vi "CRYProject Editor.vi"() -> ()   [LabVIEW 2013]
uses:
  <vilib>/Utility/miscctls.llb/LVBoundsTypeDef.ctl
  <vilib>/event_ctls.llb/eventvkey.ctl
  CRYProject Editor Global.vi
  CRYStepSetup/CRYStepSetup Global.vi
  CRYWindow/SubVI/CRYMain Sub Window Global.vi
  CRYCurveLibrary/Global/CRYCurve Library Global.vi
  CRYMainGlobal.vi
  CRYSystem/Task Sequence/CRYProject Run Control Global.vi
panel:
  out "OldPos":T1
  in  "StateOut":bool
  in  "Arg1":string
  out "RecentProjectLoad":i32
  out "EditFlag":bool
  in  "TS Name":u16(ring) items=["新建序列.cry"]
  in  "Add Step":bool
  in  "Expand/Collapse":bool caption="LegendShowOnOff"
  in  "ConfigureShowOnOff":bool caption="LegendShowOnOff"
  in  "Property seq":bool
  in  "Property step":bool
  in  "TitleShowOnOff":bool
  in  "Remove":bool
  in  "Move Down":bool
  in  "Move Up":bool
  in  "bWait":bool
  in  "TS Tree1":string(tree)
  in  "StepRemove":bool
  in  "StepLoad":bool
  in  "ProjectStateChange":bool
  in  "Load":bool
  in  "SequenceUpdate":bool
  in  "AllChange":bool
  in  "Insert":bool
  in  "Close All":bool
  in  "Close":bool
  in  "New":bool
  in  "Save":bool
  in  "Open":bool
  in  "Save As":bool
  in  "stop":bool
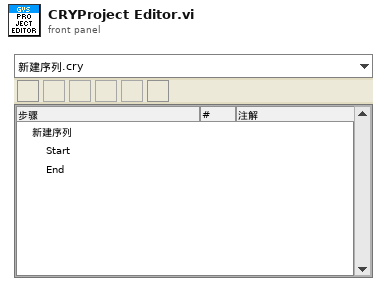
[diagram p1: front panel]
types:
  T1 = typedef "LVBoundsTypeDef.ctl" = cluster{"Width":u32, "Height":u32}
  T2 = cluster{"EventName":string, "Arg1":string, "Numeric":u16, "Numeric 2":u16, "AddSteps ":refnum<vi>, "Arg1 2":string, "Arg1 3":string, "Boolean":bool}
  T3 = typedef "eventvkey.ctl" = enum16{"ASCII", "Enter", "Return", "Shift", "Ctrl", "Alt", "Cmd", "Opt", "Caps", "NumLock", "Clear", "Break", "Up", "Down", "Left", "Right", "Insert", "Delete", "Home", "End", "PageUp", "PageDown", "Escape", "Help", "Pause", "ScrollLock", "F1", "F2", "F3", "F4", "F5", "F6", "F7", "F8", "F9", "F10", "F11", "F12", "F13", "F14", "F15", "F16", "F17", "F18", "F19", "F20", "F21", "F22", "F23", "F24", "Play", "VolumeUp", "VolumeDown", "Mute", "Two Byte Char"}
  T4 = enum16{"OK", "Yes", "YesNo", "YesNoCancel", "ReplaceAppend"}
  T5 = typedef "LVRectTypeDef.ctl" = cluster{"Left":i16, "Top":i16, "Right":i16, "Bottom":i16}
  T6 = typedef "LVPoint32TypeDef.ctl" = cluster{"Horizontal":i32, "Vertical":i32}
  T7 = typedef "CRYTS.ctl" = cluster{"No.TS":u16, "TS File Path":path, "TS Name":string, "EditStepName":string, "Steps":T8[], "New State":bool, "Change State":bool, "Flattened CurveLib Data":string, "Document Data":string, "EditStepNo":u16, "Operator Start File":string, "Sequence Type":string, "Sequence Language":string}
  T8 = typedef "CRYStep.ctl" = cluster{"No.VI":i32, "Category":string, "StepName":string, "Seq setup flattened":string, "Comment":string, "Steps config.":bool[], "Jump config":i32[], "Start":dbl, "Increment":dbl, "Name":string, "Unit":string, "Y data":u16, "Y prefix":string, "Y dB ref":dbl, "Y unit":string, "Repeat State Array":cluster{"Start":dbl, "Increment":dbl, "Count":i32, "Num":i32}[]}
  T9 = cluster{"Start":dbl, "Increment":dbl, "Count":i32, "Num":i32}[]
  T10 = cluster{"SourceRowNum":i32, "SourceCount":i32, "TargetRowNum":i32, "bResult":bool, "EditRowNum":i32}
  T11 = typedef "CRYProjectViewCluster.ctl" = cluster{"EventName":string, "Arg1":string, "Numeric":i32, "Proper VI No":i32, "AddSteps ":refnum<vi>, "Arg2":string, "Arg3":string, "Boolean":bool, "Mode":string, "Ref Variant":variant, "AllChangeFlg":bool}
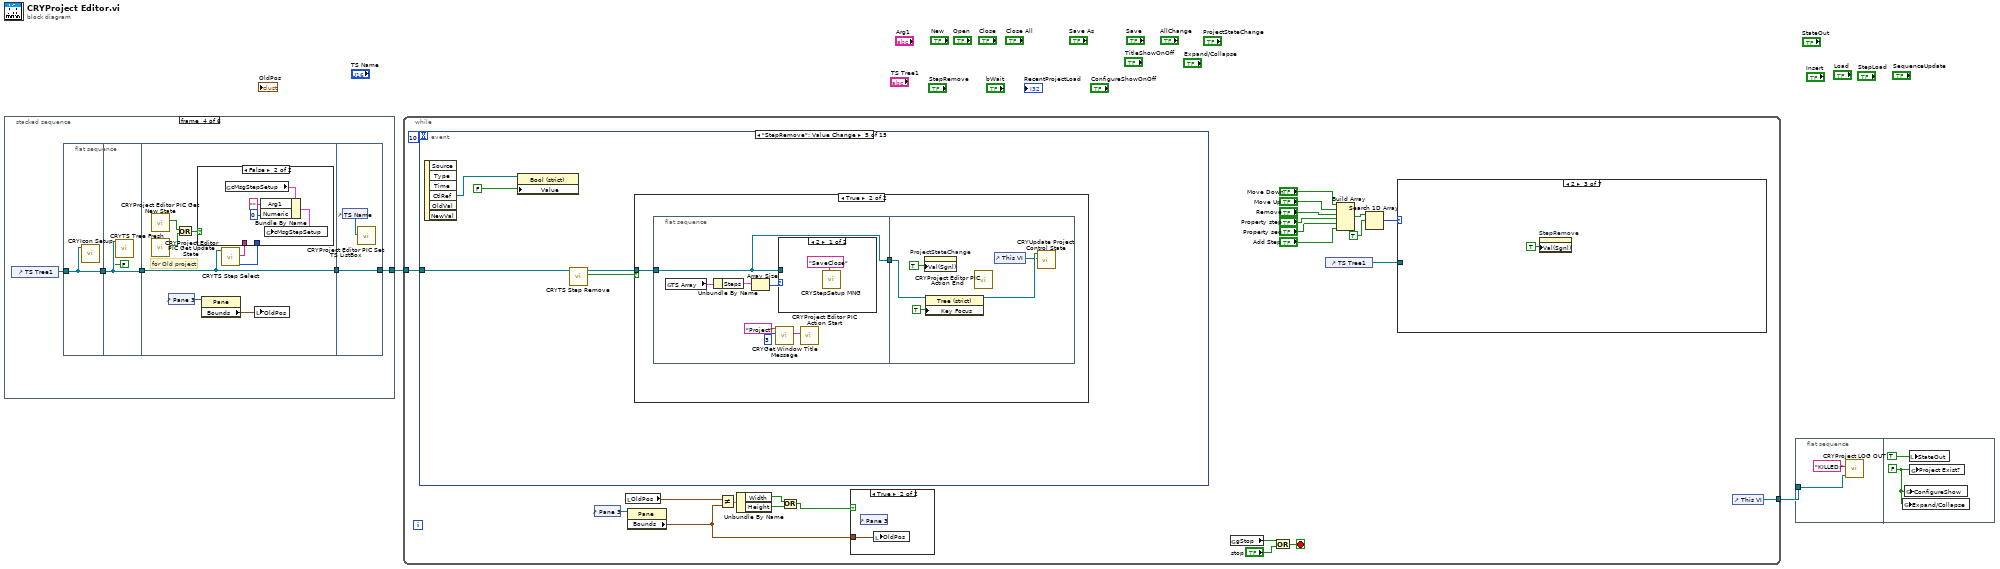
[diagram p0: block diagram]
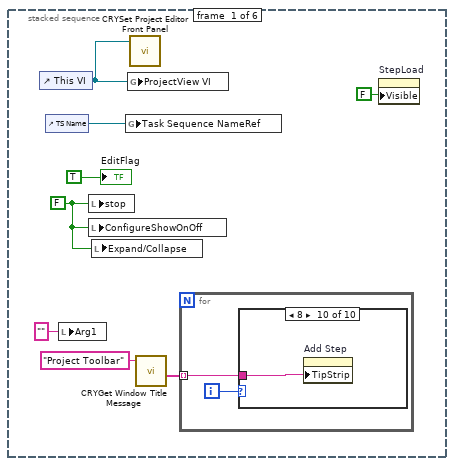
[diagram p2: hidden frame]
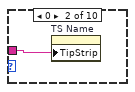
[diagram p4: hidden frame]
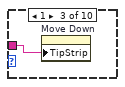
[diagram p5: hidden frame]
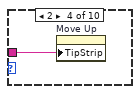
[diagram p6: hidden frame]
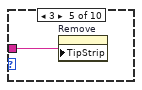
[diagram p7: hidden frame]
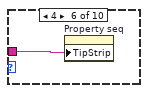
[diagram p8: hidden frame]
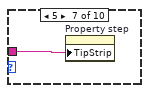
[diagram p9: hidden frame]
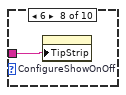
[diagram p10: hidden frame]
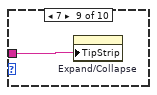
[diagram p11: hidden frame]
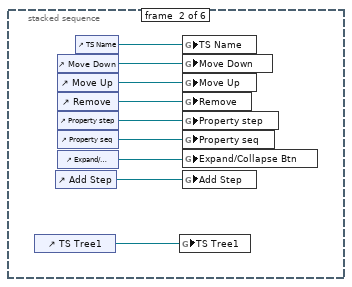
[diagram p12: hidden frame]
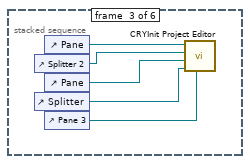
[diagram p13: hidden frame]
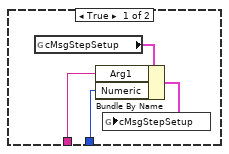
[diagram p14: hidden frame]
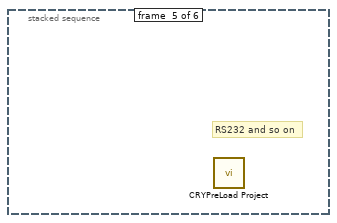
[diagram p15: hidden frame]
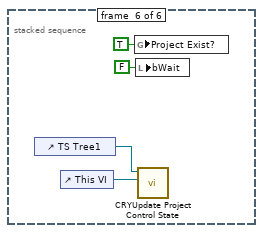
[diagram p16: hidden frame]
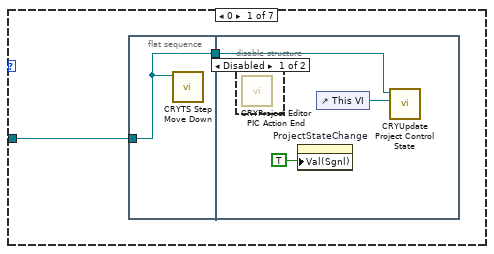
[diagram p17: hidden frame]
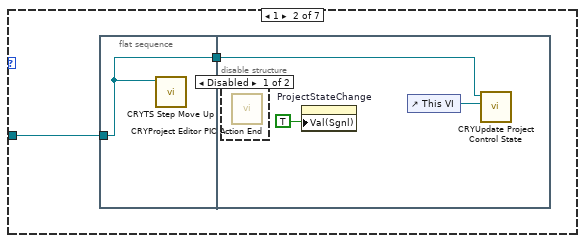
[diagram p19: hidden frame]
diagram:
  n1 = stacked-sequence {
    tunnel: [_ _ _ w36 _ _] -> w2
    frame #0 {
      w3 = FALSE ("stop")
      n2 = control-ref of="This VI"() -> (w4:refnum<vi>)
      n3 = control-ref of="TS Name"() -> (w10:refnum<vi>)
      n4 = local write "Arg1"("" ("Arg1")) -> ()
      n5 = local write "stop"(w3) -> ()
      n6 = local write "ConfigureShowOnOff"(w3) -> ()
      n7 = local write "Expand/Collapse"(w3) -> ()
      n8 = global write "CRYProject Editor Global.vi" "Task Sequence NameRef"(w10) -> ()
      n9 = global write "CRYProject Editor Global.vi" "ProjectView VI"(w4) -> ()
      n10 = call "CRYSet Project Editor Front Panel.vi"("Vi Ref"=w4) -> ()  [unwired: 11 in]
      n11 = call "CRYGet Window Title Message.vi"("Kind"="Project Toolbar") -> ("Tip Strip"=w5:string[])  [unwired: 5 in, 5 out]
      n12 = for {
        tunnel: w5 -> [w11] mode=indexing
        i -> [w12]
        n13 = case shown="8" w12 {
          tunnel: w11 -> [_ w13 w14 w15 w16 w17 w18 w19 w20 w21]
          frame Default {
          }
          frame 0 {
            n14 = property on="TS Name" class="Ring (strict)"("TipStrip"=w13) -> ()  [unwired: 2 in, 2 out]
          }
          frame 1 {
            n15 = property on="Move Down" class="Bool"("TipStrip"=w14) -> ()  [unwired: 2 in, 2 out]
          }
          frame 2 {
            n16 = property on="Move Up" class="Bool"("TipStrip"=w15) -> ()  [unwired: 2 in, 2 out]
          }
          frame 3 {
            n17 = property on="Remove" class="Bool"("TipStrip"=w16) -> ()  [unwired: 2 in, 2 out]
          }
          frame 4 {
            n18 = property on="Property seq" class="Bool"("TipStrip"=w17) -> ()  [unwired: 2 in, 2 out]
          }
          frame 5 {
            n19 = property on="Property step" class="Bool"("TipStrip"=w18) -> ()  [unwired: 2 in, 2 out]
          }
          frame 6 {
            n20 = property on="ConfigureShowOnOff" class="Bool (strict)"("TipStrip"=w19) -> ()  [unwired: 2 in, 2 out]
          }
          frame 7 {
            n21 = property on="Expand/Collapse" class="Bool (strict)"("TipStrip"=w20) -> ()  [unwired: 2 in, 2 out]
          }
          frame 8 {
            n22 = property on="Add Step" class="Bool"("TipStrip"=w21) -> ()  [unwired: 2 in, 2 out]
          }
        }
      }
      n23 = property on="StepLoad" class="Bool (strict)"("Visible"=FALSE) -> ()  [unwired: 2 in, 2 out]
      "EditFlag" <- TRUE ("EditFlag")
    }
    frame #1 {
      n24 = control-ref of="TS Tree1"() -> (w24:refnum<vi>)
      n25 = control-ref of="Add Step"() -> (w22:refnum<vi>)
      n26 = control-ref of="Move Down"() -> (w29:refnum<vi>)
      n27 = control-ref of="Move Up"() -> (w28:refnum<vi>)
      n28 = control-ref of="Remove"() -> (w27:refnum<vi>)
      n29 = control-ref of="Property step"() -> (w26:refnum<vi>)
      n30 = control-ref of="Property seq"() -> (w25:refnum<vi>)
      n31 = control-ref of="Expand/Collapse"() -> (w23:refnum<vi>)
      n32 = control-ref of="TS Name"() -> (w30:refnum<vi>)
      n33 = global write "CRYProject Editor Global.vi" "TS Tree1"(w24) -> ()
      n34 = global write "CRYProject Editor Global.vi" "TS Name"(w30) -> ()
      n35 = global write "CRYProject Editor Global.vi" "Move Down"(w29) -> ()
      n36 = global write "CRYProject Editor Global.vi" "Move Up"(w28) -> ()
      n37 = global write "CRYProject Editor Global.vi" "Remove"(w27) -> ()
      n38 = global write "CRYProject Editor Global.vi" "Property step"(w26) -> ()
      n39 = global write "CRYProject Editor Global.vi" "Property seq"(w25) -> ()
      n40 = global write "CRYProject Editor Global.vi" "Expand/Collapse Btn"(w23) -> ()
      n41 = global write "CRYProject Editor Global.vi" "Add Step"(w22) -> ()
    }
    frame #2 {
      n42 = control-ref of="Splitter 2"() -> (w34:refnum<vi>)
      n43 = control-ref of="Splitter"() -> (w32:refnum<vi>)
      n44 = control-ref of="Pane"() -> (w35:refnum<vi>)
      n45 = control-ref of="Pane"() -> (w33:refnum<vi>)
      n46 = control-ref of="Pane 3"() -> (w31:refnum<vi>)
      n47 = call "CRYInit Project Editor.vi"("Pane 3"=w31, "Splitter 2"=w32, "Pane 2"=w33, "Splitter 1"=w34, "Pane 1"=w35) -> ()  [unwired: 7 in]
    }
    frame #3 {
      n48 = control-ref of="TS Tree1"() -> (w38:refnum<vi>)
      n49 = flat-sequence {
        tunnel: w38 -> [w41]
        tunnel: [w41] -> w37
        tunnel: [w43] -> w39
        tunnel: w37 -> [w43]
        tunnel: w39 -> [w49]
        tunnel: [w49] -> w40
        tunnel: w40 -> [w61]
        tunnel: [w61] -> w36
        frame #0 {
          n50 = call "CRYIcon Setup.vi"("TS Tree In"=w41) -> ()  [unwired: 1 in, 8 out]
        }
        frame #1 {
          n51 = call "CRYTS Tree Fresh.vi"("SequenceTree"=w43, "Is Refresh?"=FALSE) -> ()  [unwired: 13 in, 1 out]
        }
        frame #2 {
          # "for Old project"
          n52 = call "CRYProject Editor PIC Get Update State.vi"() -> ("bChangeState"=w50:bool)  [unwired: 10 in, 1 out]
          n53 = call "CRYProject Editor PIC Get New State.vi"() -> ("bNewState"=w51:bool)  [unwired: 11 in]
          n54 = control-ref of="Pane 3"() -> (w45:refnum<vi>)
          n55 = Or(x=w51, y=w50) -> (x .or. y?=w48:bool)
          n56 = property class="Pane"(reference=w45) -> ("Bounds"=w44:T1)  [unwired: 1 in, 2 out]
          n57 = call "CRYTS Step Select.vi"("Tree reference In"=w49) -> ("nData_Out"=w46:i32, "sData_Out"=w47:string)  [unwired: 9 out]
          n58 = case shown="False" w48 {
            tunnel: w47 -> [w54 _]
            tunnel: w46 -> [w53 _]
            frame True {
              n59 = global read "CRYStepSetup Global.vi" "cMsgStepSetup"() -> (w55:T2)
              n60 = Bundle By Name(cluster=w55, "Arg1"=w54, "Numeric"=w53) -> (w52:T2)
              n61 = global write "CRYStepSetup Global.vi" "cMsgStepSetup"(w52) -> ()
            }
            frame False {
              n62 = global read "CRYStepSetup Global.vi" "cMsgStepSetup"() -> (w59:T2)
              n63 = Bundle By Name(cluster=w59, "Arg1"="", "Numeric"=u16 0) -> (w58:T2)
              n64 = global write "CRYStepSetup Global.vi" "cMsgStepSetup"(w58) -> ()
            }
          }
          n65 = local write "OldPos"(w44) -> ()
        }
        frame #3 {
          n66 = control-ref of="TS Name"() -> (w60:refnum<vi>)
          n67 = call "CRYProject Editor PIC Set TS ListBox.vi"("pRefTSListBox"=w60) -> ()  [unwired: 10 in, 1 out]
        }
      }
    }
    frame #4 {
      # "RS232 and so on"
      n68 = call "CRYPreLoad Project.vi"() -> ()  [unwired: 12 in]
    }
    frame #5 {
      n69 = control-ref of="TS Tree1"() -> (w62:refnum<vi>)
      n70 = control-ref of="This VI"() -> (w63:refnum<vi>)
      n71 = global write "CRYProject Editor Global.vi" "Project Exist?"(TRUE ("Project Exist?")) -> ()
      n72 = local write "bWait"(FALSE ("TreatingFlg")) -> ()
      n73 = call "CRYUpdate Project Control State.vi"("VI Ref"=w63, "RefTree In"=w62) -> ()  [unwired: 8 in, 2 out]
    }
  }
  n74 = while {
    tunnel: w2 -> [w88]
    tunnel: [w83] -> w1
    stop <- w84 stop-if-true
    n75 = event shown="[4] \"StepRemove\": Value Change" {
      selector: _ -> [_ _ _ _ _ _ _ _ _ _ _ _ _ _ _]
      dyn-events: _ -> [_ _ _ _ _ _ _ _ _ _ _ _ _ _ _]
      timeout: 10 -> [_ _ _ _ _ _ _ _ _ _ _ _ _ _ _]
      tunnel: w88 -> [_ w115 _ w133 w213 w240 w258 w264 w291 w296 w314 w316 w320 _ w356]
      event Timeout {
        n76 = event-data() -> ()  [unwired: 3 out]
      }
      event Pane Size {
        n77 = event-data() -> ("NewBnds"=w119:T5)  [unwired: 5 out]
        n78 = Unbundle By Name(w119) -> ("Right"=w118:i16, "Left"=w117:i16)  [unwired: 2 out]
        n79 = control-ref of="Splitter 2"() -> (w111:refnum<vi>)
        n80 = control-ref of="Splitter"() -> (w113:refnum<vi>)
        n81 = control-ref of="Pane"() -> (w110:refnum<vi>)
        n82 = control-ref of="Pane"() -> (w112:refnum<vi>)
        n83 = control-ref of="Pane 3"() -> (w114:refnum<vi>)
        n84 = Subtract(x=w118, y=w117) -> (x-y=w116:i16)
        n85 = call "CRYInit Project Editor.vi"("Pane 3"=w114, "Splitter 2"=w113, "Pane 2"=w112, "Splitter 1"=w111, "Pane 1"=w110) -> ()  [unwired: 7 in]
        n86 = disable-structure shown="Disabled" {
          disable-tunnel: w116 -> [w122 _]
          disable-tunnel: w115 -> [w120 _]
          frame Disabled {
            n87 = property on="Property Node" class="Tree (strict)"(reference=w120, "Width"=w122, "ActiveColNum"=0 ("Active Cell:Active Column Number")) -> ()  [unwired: 1 in, 2 out]
          }
          frame Enabled {
          }
        }
      }
      event "TS Tree1": Shortcut Menu Activation? {
        n88 = event-data() -> ("CtlRef"=w123:refnum<vi>, "MenuRef"=w128:refnum<k9>, "Coords"=w125:T6)  [unwired: 5 out]
        n89 = call "CRYGet Tree Click State.vi"("Coords"=w125, "Tree Ref In"=w123) -> ("Tag"=w124:string)  [unwired: 9 out]
        n90 = Not Equal?(x=w124, y="") -> (x != y?=w126:bool)
        n91 = case shown="True" w126 {
          tunnel: w128 -> [_ w132]
          tunnel: w123 -> [_ w130]
          tunnel: w125 -> [_ w131]
          frame False {
          }
          frame True {
            n92 = control-ref of="This VI"() -> (w129:refnum<vi>)
            n93 = call "CRYProject Popup Menu.vi"("Tree Reference In"=w130, "Coords In"=w131, "This VI"=w129, "Menu Ref In"=w132) -> ()  [unwired: 8 out]
          }
        }
        n94 = event-data() -> ()  [unwired: 1 in, 2 out]
      }
      event "TS Tree1": Shortcut Menu Selection (User) {
        n95 = event-data() -> ("CtlRef"=w134:refnum<vi>, "ItemTag"=w136:string, "Coords"=w135:T6)  [unwired: 6 out]
        n96 = case shown="\"STEP_RENAME\"" w136 {
          tunnel: w135 -> [_ _ w138 _ _ _ _]
          tunnel: w134 -> [_ w137 w139 _ _ _ w164]
          tunnel: w133 -> [_ _ _ w143 w146 _ _]
          frame "", Default {
          }
          frame "OPEN_SEQUENCE_CONFIGURE" {
            n97 = call "CRYStart Editor.vi"("Project Tree reference"=w137) -> ()  [unwired: 10 in, 1 out]
          }
          frame "OPEN_STEP_CONFIGURE" {
            n98 = call "CRYGet Tree Click State.vi"("Coords"=w138, "Tree Ref In"=w139) -> ()  [unwired: 10 out]
            n99 = call "CRYProject Tree Action Check.vi"("sOption"="Configure", "Project Tree reference"=w139) -> ("bResult"=w140:bool)  [unwired: 8 in, 1 out]
            n100 = case shown="True" w140 {
              tunnel: w139 -> [_ w142]
              frame False {
              }
              frame True {
                n101 = call "CRYConfigure Step.vi"("Project Tree reference"=w142) -> ()  [unwired: 10 in, 1 out]
              }
            }
          }
          frame "STEP_MOVE_DOWN" {
            n102 = flat-sequence {
              tunnel: w143 -> [w144]
              frame #0 {
                n103 = call "CRYTS Step Move Down.vi"("Sequence"=w144) -> ()  [unwired: 1 in, 10 out]
              }
              frame #1 {
                n104 = property on="ProjectStateChange" class="Bool (strict)"("Val(Sgnl)"=TRUE ("Value (Signaling)")) -> ()  [unwired: 2 in, 2 out]
              }
            }
          }
          frame "STEP_MOVE_UP" {
            n105 = flat-sequence {
              tunnel: w146 -> [w147]
              frame #0 {
                n106 = call "CRYTS Step Move Up.vi"("TreeRefereneIn"=w147) -> ()  [unwired: 1 in, 10 out]
              }
              frame #1 {
                n107 = property on="ProjectStateChange" class="Bool (strict)"("Val(Sgnl)"=TRUE ("Value (Signaling)")) -> ()  [unwired: 2 in, 2 out]
              }
            }
          }
          frame "STEP_DELETE" {
            n108 = property on="StepRemove" class="Bool (strict)"("Val(Sgnl)"=TRUE ("Value (Signaling)")) -> ()  [unwired: 2 in, 2 out]
          }
          frame "STEP_RENAME" {
            n109 = property on="Property Node" class="Tree (strict)"(reference=w164) -> (reference out=w168:refnum<vi>, "Value"=w163:string)  [unwired: 1 in, 1 out]
            n110 = global read "CRYProject Editor Global.vi" "TS Array"() -> (w157:T7)
            n111 = call "CRYGet Tree Step No.vi"("SequenceTree"=w164, "Active Item Tag"=w163) -> ("Active Cell String4"=w165:string)  [unwired: 12 in, 1 out]
            n112 = Decimal String To Number(string=w165) -> (number=w159:i32)  [unwired: 2 in, 1 out]
            n113 = Unbundle By Name(w157) -> ("Steps"=w156:T8[])
            n114 = property class="Tree (strict)"(reference=w168, "Active Item Tag"=w163, "ActiveColNum"=0 ("Active Cell:Active Column Number")) -> (reference out=w166:refnum<vi>, "Cell String"=w153:string)  [unwired: 1 in, 1 out]
            n115 = Index Array(array=w156, index=w159) -> (element=w158:T8)
            n116 = Unbundle By Name(w158) -> ("Repeat State Array"=w162:T9)
            n117 = Array Size(array=w162) -> (size(s)=w160:i32)
            n118 = for {
              N: w160 -> [_]
              shift-right: [w173] -> w151
              shift-left: "" ("decimal integer string") -> [w172]
              n119 = Concatenate Strings(w172, "     " ("decimal integer string")) -> (w173:string)
            }
            n120 = Match Pattern(string=w153, regular expression=w151) -> (before substring=w155:string, after substring=w154:string)  [unwired: 1 in, 2 out]
            n121 = Empty String/Path?(string/path=w155) -> (empty?=w150:bool)
            n122 = Select(t=w154, s=w150, f=w153) -> (s? t:f=w152:string)
            n123 = call "CRYGet Step Name Dialog.vi"("Step Name"=w152) -> ("Step Name Out"=w170:string, "Return Flag"=w169:bool)  [unwired: 9 in]
            n124 = case shown="True" w169 {
              tunnel: w166 -> [_ w187]
              tunnel: w170 -> [_ w176]
              tunnel: w163 -> [_ w186]
              tunnel: w159 -> [_ w185]
              tunnel: w158 -> [_ w184]
              tunnel: w157 -> [_ w182]
              tunnel: w156 -> [_ w183]
              tunnel: w150 -> [_ w181]
              tunnel: w151 -> [_ w180]
              frame False {
              }
              frame True {
                n125 = Select(t=w180, s=w181, f="") -> (s? t:f=w177:string)
                n126 = Concatenate Strings(w177, w176) -> (w178:string)
                n127 = flat-sequence {
                  tunnel: w187 -> [w201]
                  tunnel: w186 -> [w200]
                  tunnel: w185 -> [w191]
                  tunnel: w184 -> [w198]
                  tunnel: w183 -> [w197]
                  tunnel: w182 -> [w196]
                  tunnel: w178 -> [w195]
                  tunnel: w176 -> [w192]
                  tunnel: [w191] -> w175
                  tunnel: [w188] -> w174
                  tunnel: w175 -> [w209]
                  tunnel: w174 -> [w205]
                  frame #0 {
                    n128 = global read "CRYStepSetup Global.vi" "Step Setup Exist"() -> (w194:bool)
                    n129 = global read "CRYStepSetup Global.vi" "Step SubVI Ref"() -> (w193:refnum<vi>)
                    n130 = Bundle By Name(cluster=w198, "StepName"=w192) -> (w189:T8)
                    n131 = property class="Tree (strict)"(reference=w201, "Active Item Tag"=w200, "ActiveColNum"=0 ("Active Cell:Active Column Number"), "Cell String"=w195) -> ()  [unwired: 1 in, 2 out]
                    n132 = case shown="True" w194 {
                      tunnel: w193 -> [_ w204]
                      tunnel: w192 -> [_ w203]
                      frame False {
                      }
                      frame True {
                        n133 = property class="VI"(reference=w204, "Front Panel.Title"=w203) -> ()  [unwired: 1 in, 2 out]
                      }
                    }
                    n134 = Replace Array Subset(array=w197, new element=w189, index=w191) -> (w190:T8[])
                    n135 = Bundle By Name(cluster=w196, "Steps"=w190) -> (w199:T7)
                    n136 = global write "CRYProject Editor Global.vi" "TS Array"(w199) -> ()
                    n137 = Unbundle By Name(w189) -> ("No.VI"=w188:i32)
                  }
                  frame #1 {
                    n138 = global read "CRYCurve Library Global.vi" "Curve Library VI"() -> (w208:refnum<vi>)
                    n139 = call "CRYRename Data by Step Rename.vi"("Tree VI No."=w209) -> ()  [unwired: 11 in]
                    n140 = property on="ProjectStateChange" class="Bool (strict)"("Val(Sgnl)"=TRUE ("Value (Signaling)")) -> ()  [unwired: 2 in, 2 out]
                    n141 = call "CRYGet Numeric Reference.vi"("Label Name"="StepNameChange", "VI Refnum"=w208) -> ("Numeric Ref Out"=w206:refnum<vi>)  [unwired: 7 in, 2 out]
                    n142 = property class="DigNum"(reference=w206, "Val(Sgnl)"=w205) -> ()  [unwired: 1 in, 2 out]
                  }
                }
              }
            }
          }
        }
      }
      event "StepRemove": Value Change {
        n143 = event-data() -> ("CtlRef"=w214:refnum<vi>)  [unwired: 6 out]
        n144 = property on="Property Node" class="Bool (strict)"(reference=w214, "Value"=FALSE ("Remove")) -> ()  [unwired: 1 in, 2 out]
        n145 = call "CRYTS Step Remove.vi"("Tree Sequence"=w213) -> ("bResult"=w212:bool, "Tree Sequence Ref Out"=w211:refnum<vi>)  [unwired: 2 in, 7 out]
        n146 = case shown="True" w212 {
          tunnel: w211 -> [w218 w221]
          frame False {
            n147 = property class="Tree (strict)"(reference=w218, "Key Focus"=TRUE) -> (reference out=w216:refnum<vi>)  [unwired: 1 in, 1 out]
            n148 = control-ref of="This VI"() -> (w217:refnum<vi>)
            n149 = call "CRYUpdate Project Control State.vi"("VI Ref"=w217, "RefTree In"=w216) -> ()  [unwired: 8 in, 2 out]
          }
          frame True {
            n150 = flat-sequence {
              tunnel: w221 -> [w225]
              tunnel: [w225] -> w220
              tunnel: w220 -> [w234]
              frame #0 {
                n151 = global read "CRYProject Editor Global.vi" "TS Array"() -> (w223:T7)
                n152 = Unbundle By Name(w223) -> ("Steps"=w224:T8[])
                n153 = Array Size(array=w224) -> (size(s)=w222:i32)
                n154 = call "CRYGet Window Title Message.vi"("No"=3 ("Error No"), "Kind"="Project") -> ("Unicode String"=w227:string)  [unwired: 4 in, 5 out]
                n155 = case shown="2" w222 {
                  tunnel: w225 -> [_ w231]
                  frame 2 {
                    n156 = call "CRYStepSetup MNG.vi"("sAction"="SaveClose") -> ()  [unwired: 9 in, 2 out]
                  }
                  frame Default {
                    n157 = call "CRYTS Step Select.vi"("Tree reference In"=w231) -> ("nData_Out"=w232:i32, "sData_Out"=w233:string)  [unwired: 9 out]
                    n158 = call "CRYStep Setup Replace.vi"("sOption Etc"="StepRemove" ("sOption"), "Current Step Setup VI No"=w232, "Category"=w233) -> ()  [unwired: 1 in, 8 out]
                  }
                }
                n159 = call "CRYProject Editor PIC Action Start.vi"("sData"=w227) -> ()  [unwired: 11 in]
              }
              frame #1 {
                n160 = property on="ProjectStateChange" class="Bool (strict)"("Val(Sgnl)"=TRUE ("Value (Signaling)")) -> ()  [unwired: 2 in, 2 out]
                n161 = property class="Tree (strict)"(reference=w234, "Key Focus"=TRUE) -> (reference out=w238:refnum<vi>)  [unwired: 1 in, 1 out]
                n162 = call "CRYProject Editor PIC Action End.vi"() -> ()  [unwired: 12 in]
                n163 = control-ref of="This VI"() -> (w237:refnum<vi>)
                n164 = call "CRYUpdate Project Control State.vi"("VI Ref"=w237, "RefTree In"=w238) -> ()  [unwired: 8 in, 2 out]
              }
            }
          }
        }
      }
      event "Expand/Collapse": Value Change {
        n165 = event-data() -> ("NewVal"=w239:bool)  [unwired: 6 out]
        n166 = flat-sequence {
          tunnel: [w245] -> w243
          tunnel: w240 -> [w245]
          tunnel: w239 -> [w244]
          tunnel: [w250] -> w242
          tunnel: [w248] -> w241
          tunnel: w243 -> [w246]
          tunnel: w242 -> [w252]
          tunnel: w241 -> [w251]
          frame #0 {
            n167 = global write "CRYProject Editor Global.vi" "Expand/Collapse"(w244) -> ()
          }
          frame #1 {
            n168 = call "CRYCalculation TS Tree RowNum.vi"("Tree Task SequenceIn"=w246, "sOption"="Step Configure") -> ("DispInfo Cluster Out"=w249:T10, "Tree Task Sequence Out"=w250:refnum<vi>)  [unwired: 7 in, 5 out]
            n169 = Unbundle By Name(w249) -> ("EditRowNum"=w248:i32)
          }
          frame #2 {
            n170 = call "CRYTS Tree Fresh.vi"("SequenceTree"=w252, "Edit Index"=w251, "Is Refresh?"=FALSE) -> ()  [unwired: 12 in, 1 out]
          }
        }
      }
      event "Save As": Value Change {
        w259 = 0 ("Active Cell:Active Column Number")
        n171 = event-data() -> ()  [unwired: 7 out]
        n172 = control-ref of="TS Name"() -> (w261:refnum<vi>)
        n173 = property on="Property Node" class="Tree (strict)"(reference=w258, "Active Item Row Number"=w259, "ActiveColNum"=w259) -> (reference out=w260:refnum<vi>, "Active Item Tag"=w254:string)  [unwired: 1 in, 1 out]
        n174 = call "CRYProject Editor PIC Set TS ListBox.vi"("pRefTSListBox"=w261) -> ("TS Name Out"=w256:string)  [unwired: 10 in]
        n175 = Match Pattern(string=w256, regular expression=".cry") -> (before substring=w255:string)  [unwired: 1 in, 3 out]
        n176 = property on="Property Node" class="Tree (strict)"(reference=w260, "Active Item Tag"=w254, "Cell String"=w255) -> ()  [unwired: 1 in, 2 out]
      }
      event "TS Tree1": Double Click {
        n177 = event-data() -> ("Coords"=w263:T6, "Tag"=w265:string)  [unwired: 8 out]
        n178 = call "CRYGet Tree Click State.vi"("Coords"=w263, "Tree Ref In"=w264) -> ("In Bounds?"=w262:bool)  [unwired: 4 in, 5 out]
        n179 = case shown="True" w262 {
          tunnel: w265 -> [_ w268]
          tunnel: w264 -> [_ w267]
          tunnel: w263 -> [_ w266]
          frame False {
          }
          frame True {
            n180 = flat-sequence {
              tunnel: w267 -> [w273]
              tunnel: [w273] -> w271
              tunnel: [w275] -> w270
              tunnel: w266 -> [w275]
              tunnel: w268 -> [w274]
              tunnel: [w274] -> w269
              tunnel: w271 -> [w279]
              tunnel: w270 -> [w281]
              tunnel: w269 -> [w278]
              frame #0 {
                n181 = global read "CRYMainGlobal.vi" "Access Level"() -> (w272:enum16{"Engineer", "Technician", "Operator"})
                n182 = case shown="\"Engineer\"" w272 {
                  tunnel: w273 -> [w276 _]
                  frame "Engineer" {
                    n183 = control-ref of="This VI"() -> (w277:refnum<vi>)
                    n184 = call "CRYUpdate Project Control State.vi"("VI Ref"=w277, "RefTree In"=w276) -> ()  [unwired: 8 in, 2 out]
                  }
                  frame "Operator", Default {
                  }
                }
              }
              frame #1 {
                n185 = call "CRYProject Tree Action Check.vi"("tag"=w278, "Coords In"=w281, "sOption"="Tree DblClick", "Project Tree reference"=w279) -> ("Type Out"=w280:string, "bResult"=w282:bool)  [unwired: 6 in]
                n186 = case shown="True" w282 {
                  tunnel: w280 -> [_ w285]
                  tunnel: w279 -> [_ w284]
                  frame False {
                  }
                  frame True {
                    n187 = case shown="\"main\"" w285 {
                      tunnel: w284 -> [_ w286 w287 _]
                      frame Default {
                      }
                      frame "Seq Config" {
                        n188 = call "CRYStart Editor.vi"("Project Tree reference"=w286) -> ()  [unwired: 10 in, 1 out]
                      }
                      frame "Step Config" {
                        n189 = call "CRYConfigure Step.vi"("Project Tree reference"=w287) -> ()  [unwired: 10 in, 1 out]
                      }
                      frame "main" {
                        n190 = call "CRYPreUpdate Sequence.vi"("EventName"="StepLoadFromProject", "AllChangeFlg"=TRUE) -> ()  [unwired: 14 in]
                      }
                    }
                  }
                }
              }
            }
          }
        }
      }
      event "TS Tree1": Mouse Down {
        n191 = event-data() -> ()  [unwired: 9 out]
        n192 = global read "CRYMainGlobal.vi" "Access Level"() -> (w290:enum16{"Engineer", "Technician", "Operator"})
        n193 = case shown="\"Technician\", Default" w290 {
          tunnel: w291 -> [w292 _]
          frame "Engineer" {
            n194 = control-ref of="This VI"() -> (w293:refnum<vi>)
            n195 = call "CRYUpdate Project Control State.vi"("VI Ref"=w293, "RefTree In"=w292) -> ()  [unwired: 8 in, 2 out]
            n196 = local write "EditFlag"(TRUE ("EditFlag")) -> ()
          }
          frame "Technician", Default {
          }
        }
      }
      event "TS Tree1": Key Down {
        n197 = event-data() -> ("VKey"=w297:T3)  [unwired: 10 out]
        n198 = global read "CRYMainGlobal.vi" "Access Level"() -> (w295:enum16{"Engineer", "Technician", "Operator"})
        n199 = case shown="\"Technician\", Default" w295 {
          tunnel: w297 -> [w299 _]
          tunnel: w296 -> [w298 _]
          frame "Engineer" {
            n200 = flat-sequence {
              tunnel: w299 -> [w303]
              tunnel: [w303] -> w300
              tunnel: w298 -> [w302]
              tunnel: w300 -> [w306]
              frame #0 {
                n201 = control-ref of="This VI"() -> (w301:refnum<vi>)
                n202 = call "CRYUpdate Project Control State.vi"("VI Ref"=w301, "RefTree In"=w302) -> ()  [unwired: 8 in, 2 out]
              }
              frame #1 {
                n203 = Equal?(x=w306, y=eventvkey."Delete" ("VKey")) -> (x = y?=w304:bool)
                n204 = case shown="True" w304 {
                  frame False {
                  }
                  frame True {
                    n205 = property on="StepRemove" class="Bool (strict)"("Val(Sgnl)"=TRUE ("Value (Signaling)")) -> ()  [unwired: 2 in, 2 out]
                  }
                }
              }
            }
          }
          frame "Technician", Default {
            n206 = call "CRYGet Error Message.vi"("Kind"="Step Setup") -> ("Window Title"=w310:string)  [unwired: 5 in, 5 out]
            n207 = call "CRYGet Access Level Message.vi"() -> ("Multibyte string"=w308:string)  [unwired: 11 in]
            n208 = call "CRYMessage Dialog.vi"("Window Title"=w310, "YesNoCancel"=T4."OK", "Message Content"=w308) -> ()  [unwired: 7 in, 2 out]
          }
        }
      }
      event "TS Tree1": event type 3.0.x80000011; "TS Tree1": Item Open? {
        n209 = event-data() -> ("Tag"=w315:string)  [unwired: 5 out]
        n210 = invoke class="Tree (strict)" method="Double Click"(reference=w314) -> ("Double Click"=w313:string)  [unwired: 2 in, 2 out]
        n211 = Equal?(x=w315, y=w313) -> (x = y?=w312:bool)
        n212 = event-data("Discard?"=w312) -> ()  [unwired: 1 in, 1 out]
      }
      event "TS Tree1": event #0x1e; "TS Tree1": Item Close {
        n213 = event-data() -> ()  [unwired: 6 out]
        n214 = control-ref of="This VI"() -> (w317:refnum<vi>)
        n215 = local write "EditFlag"(FALSE ("EditFlag")) -> ()
        n216 = call "CRYUpdate Project Control State.vi"("VI Ref"=w317, "RefTree In"=w316) -> ()  [unwired: 8 in, 2 out]
      }
      event "TS Name": Value Change {
        n217 = event-data() -> ("CtlRef"=w322:refnum<vi>, "OldVal"=w319:u16)  [unwired: 5 out]
        n218 = property on="TS Name" class="Ring (strict)"() -> ("RingText.Text"=w323:string)  [unwired: 2 in, 2 out]
        n219 = flat-sequence {
          tunnel: w319 -> [w326]
          tunnel: w323 -> [w328]
          tunnel: [w328] -> w321
          tunnel: w322 -> [w327]
          tunnel: w320 -> [w324]
          tunnel: w321 -> [w329]
          frame #0 {
            n220 = property class="Ring (strict)"(reference=w327, "Value"=w326) -> ()  [unwired: 1 in, 2 out]
            n221 = control-ref of="This VI"() -> (w325:refnum<vi>)
            n222 = call "CRYUpdate Project Control State.vi"("VI Ref"=w325, "RefTree In"=w324) -> ()  [unwired: 8 in, 2 out]
          }
          frame #1 {
            n223 = global read "CRYProject Editor Global.vi" "TS Array"() -> (w331:T7)
            n224 = Unbundle By Name(w331) -> ("TS File Path"=w333:path)
            n225 = Path To String(path=w333) -> (string=w334:string)
            n226 = Concatenate Strings(w334, "\\" ("string"), w329) -> (w332:string)
            n227 = call "CRYProject Editor PIC Send Event to Main.vi"("nData"=0, "sData"=w332, "sEventName"="OpenProjectFullPath") -> ()  [unwired: 9 in]
          }
          frame #2 {
            n228 = call "CRYProject Editor PIC Action End.vi"() -> ()  [unwired: 12 in]
          }
        }
      }
      event "ProjectStateChange": Value Change {
        n229 = event-data() -> ()  [unwired: 7 out]
        n230 = global read "CRYProject Editor Global.vi" "bProjectLoaded"() -> (w342:bool)
        n231 = global read "CRYMainGlobal.vi" "Sequence Generator"() -> (w338:bool)
        n232 = global read "CRYProject Run Control Global.vi" "RunState"() -> (w341:bool)
        n233 = global read "CRYMainGlobal.vi" "Quick Lunch"() -> (w339:bool)
        n234 = Or(x=w339, y=w338) -> (x .or. y?=w337:bool)
        n235 = Compound Arithmetic op=AND(w342, invert w341, invert w337) -> (w340:bool)
        n236 = case shown="True" w340 {
          frame False {
          }
          frame True {
            n237 = global read "CRYProject Editor Global.vi" "TS Array"() -> (w345:T7)
            n238 = Unbundle By Name(w345) -> ("Change State"=w344:bool)
            n239 = case shown="False" w344 {
              selector: w344 -> [w352 w353]
              tunnel: [w352 w353] -> w343
              frame True {
              }
              frame False {
                n240 = call "CRYProject Editor PIC Change State.vi"("bChangeState"=TRUE ("Change State")) -> ()  [unwired: 11 in]
              }
            }
            n241 = flat-sequence {
              tunnel: w343 -> [_]
              frame #0 {
                n242 = global read "CRYMain Sub Window Global.vi" "Main Menu Refnum"() -> (w349:refnum<k9>)
                n243 = call "CRYMenu Language Set.vi"("sID"="FILE_SAVE") -> ("sMultibyte_Out"=w350:string, "sID_Out"=w351:string)  [unwired: 7 in, 2 out]
                n244 = Set Menu Item Info(6:FALSE ("checked"), 7:w351, 9:TRUE ("enabled"), 10:w350, 11:w349) -> ()  [unwired: 1 in, 3 out]
              }
            }
          }
        }
      }
      event "AllChange": Value Change {
        n245 = event-data() -> ()  [unwired: 7 out]
        n246 = local read "bWait"() -> (w355:bool)
        n247 = case shown="False" w355 {
          tunnel: w356 -> [w362 _]
          frame False {
            n248 = flat-sequence {
              tunnel: w362 -> [w366]
              tunnel: [w366] -> w361
              tunnel: [w372] -> w364
              tunnel: [w371] -> w363
              tunnel: w361 -> [w370]
              tunnel: [w369] -> w358
              tunnel: [w368] -> w357
              tunnel: w364 -> [w517]
              tunnel: w363 -> [w520]
              tunnel: [w517] -> w360
              tunnel: [w516] -> w359
              tunnel: w358 -> [_]
              tunnel: w357 -> [_]
              tunnel: w360 -> [w530]
              tunnel: w359 -> [w529]
              frame #0 {
                n249 = local write "bWait"(TRUE ("Project Exist?")) -> ()
              }
              frame #1 {
                n250 = call "CRYPull Data From ProjectViewCluster Array.vi"() -> ("Is Remain ?"=w372:bool, "ProjectViewCluster Out"=w371:T11)  [unwired: 10 in]
                n251 = global read "CRYMainGlobal.vi" "Access Level"() -> (w367:enum16{"Engineer", "Technician", "Operator"})
                n252 = Unbundle By Name(w371) -> ("EventName"=w368:string, "Arg1"=w374:string, "Proper VI No"=w373:i32)
                n253 = case shown="\"StepLoadFromProject\"" w368 {
                  tunnel: w370 -> [w375 w379 w388 w394 w406 w424 w441 w479 w480 w481 w482 w483 w490 w504]
                  tunnel: w374 -> [_ _ _ _ _ _ w437 _ _ _ _ w485 _ _]
                  tunnel: w373 -> [_ _ _ _ _ _ w438 _ _ _ _ w484 _ _]
                  tunnel: w371 -> [_ w378 w387 w396 w404 _ _ w478 _ _ _ _ w489 w513]
                  tunnel: w367 -> [_ _ _ _ _ w423 w440 _ _ _ _ _ _ _]
                  tunnel: [w375 w376 w386 w394 w403 w422 w439 w476 w480 w481 w482 w483 w486 w504] -> w369
                  frame "", Default {
                  }
                  frame "Insert Step" {
                    n254 = flat-sequence {
                      tunnel: w379 -> [w382]
                      tunnel: w378 -> [w381]
                      tunnel: [w380] -> w377
                      tunnel: [w384] -> w376
                      tunnel: w377 -> [w384]
                      frame #0 {
                        n255 = Unbundle By Name(w381) -> ("AddSteps"=w383:refnum<vi>)
                        n256 = call "CRYTS Step Insert.vi"("Steps"=w383, "Tree Task SequenceIn"=w382) -> ("Tree Task Sequence Out"=w380:refnum<vi>)  [unwired: 1 in, 8 out]
                      }
                      frame #1 {
                        n257 = call "CRYProject Editor PIC Action End.vi"() -> ()  [unwired: 12 in]
                      }
                    }
                  }
                  frame "Insert Sequence" {
                    n258 = flat-sequence {
                      tunnel: w388 -> [w391]
                      tunnel: w387 -> [w392]
                      tunnel: [w389] -> w385
                      tunnel: [w393] -> w386
                      tunnel: w385 -> [w393]
                      frame #0 {
                        n259 = Unbundle By Name(w392) -> ("AddSteps"=w390:refnum<vi>)
                        n260 = call "CRYTS Sequence Insert.vi"("Steps"=w390, "Tree Task SequenceIn"=w391) -> ("Tree Task Sequence Out"=w389:refnum<vi>)  [unwired: 9 in]
                      }
                      frame #1 {
                        n261 = call "CRYProject Editor PIC Action End.vi"() -> ()  [unwired: 12 in]
                      }
                    }
                  }
                  frame "SequenceUpdate" {
                    n262 = Unbundle By Name(w396) -> ("Arg1"=w400:string, "Proper VI No"=w399:i32, "Arg2"=w398:string, "Arg3"=w397:string)
                    n263 = call "CRYStep Update.vi"("SequenceTree"=w394, "StepName"=w397, "Step Name Write"=FALSE ("Name/Identifier"), "Seq-step setup"=w398, "Proper VI No"=w399, "StepIdentifier"=w400) -> ()  [unwired: 1 in, 5 out]
                  }
                  frame "Load" {
                    n264 = flat-sequence {
                      tunnel: w406 -> [w412]
                      tunnel: [w413] -> w405
                      tunnel: w404 -> [w413]
                      tunnel: [w410] -> w401
                      tunnel: w405 -> [w416]
                      tunnel: [w414] -> w402
                      tunnel: w401 -> [w414]
                      tunnel: [w421] -> w403
                      tunnel: w402 -> [w421]
                      frame #0 {
                        n265 = call "CRYUpdate Tree for Load.vi"("Is Move?"=FALSE, "ProjectViewCluster In"=w413, "RefTree In"=w412) -> ("RefTree Out"=w410:refnum<vi>)  [unwired: 8 in]
                      }
                      frame #1 {
                        n266 = Unbundle By Name(w416) -> ("Arg1"=w420:string, "Proper VI No"=w419:i32, "Arg2"=w418:string, "Arg3"=w417:string)
                        n267 = call "CRYStep Update.vi"("StepName"=w417, "Step Name Write"=TRUE ("Name/Identifier"), "Seq-step setup"=w418, "Proper VI No"=w419, "StepIdentifier"=w420) -> ()  [unwired: 2 in, 5 out]
                      }
                      frame #2 {
                        n268 = call "CRYProject Editor PIC Action End.vi"() -> ()  [unwired: 12 in]
                      }
                    }
                    n269 = disable-structure shown="Enabled" {
                      frame Disabled {
                        n270 = call "CRYGet Window Title Message.vi"("No"=1 ("Error No"), "Kind"="Project") -> ("Unicode String"=w408:string)  [unwired: 4 in, 5 out]
                        n271 = call "CRYProject Editor PIC Action Start.vi"("sData"=w408) -> ()  [unwired: 11 in]
                      }
                      frame Enabled {
                      }
                    }
                  }
                  frame "StepLoadFromProject" {
                    n272 = case shown="\"Engineer\", \"Technician\"" w423 {
                      tunnel: w424 -> [_ w430]
                      tunnel: [_ w429] -> w422
                      frame Default {
                        n273 = call "CRYGet Error Message.vi"("Kind"="Step Setup") -> ("Window Title"=w427:string)  [unwired: 5 in, 5 out]
                        n274 = call "CRYGet Access Level Message.vi"() -> ("Multibyte string"=w425:string)  [unwired: 11 in]
                        n275 = call "CRYMessage Dialog.vi"("Window Title"=w427, "YesNoCancel"=T4."OK", "Message Content"=w425) -> ()  [unwired: 7 in, 2 out]
                      }
                      frame "Engineer", "Technician" {
                        n276 = flat-sequence {
                          tunnel: w430 -> [w433]
                          tunnel: [w432] -> w431
                          tunnel: w431 -> [w434]
                          tunnel: [w434] -> w429
                          frame #0 {
                            n277 = call "CRYUpdate Edit Step Name.vi"("Tree reference In"=w433) -> ("reference out"=w432:refnum<vi>)  [unwired: 10 in]
                          }
                          frame #1 {
                            n278 = call "CRYTS Step Select.vi"("Tree reference In"=w434) -> ("nData_Out"=w436:i32, "sData_Out"=w435:string)  [unwired: 9 out]
                            n279 = call "CRYStep Setup Replace.vi"("Current Step Setup VI No"=w436, "Category"=w435) -> ()  [unwired: 2 in, 8 out]
                          }
                          frame #2 {
                            n280 = call "CRYProject Editor PIC Action End.vi"() -> ()  [unwired: 12 in]
                          }
                        }
                      }
                    }
                  }
                  frame "StepLoadFromToolbar" {
                    n281 = case shown="\"Engineer\", \"Technician\"" w440 {
                      tunnel: w441 -> [_ w450]
                      tunnel: [_ w449] -> w439
                      tunnel: w438 -> [_ w448]
                      tunnel: w437 -> [_ w447]
                      frame Default {
                        n282 = call "CRYGet Error Message.vi"("Error No"=0, "Kind"="Step Setup") -> ("Message"=w445:string, "Window Title"=w444:string)  [unwired: 4 in, 4 out]
                        n283 = call "CRYMessage Dialog.vi"("Window Title"=w444, "YesNoCancel"=T4."OK", "Message Content"=w445) -> ()  [unwired: 7 in, 2 out]
                      }
                      frame "Engineer", "Technician" {
                        n284 = disable-structure shown="Enabled" {
                          disable-tunnel: w450 -> [w453 w466]
                          disable-tunnel: [w452 w465] -> w449
                          disable-tunnel: w448 -> [w451 w462]
                          disable-tunnel: w447 -> [_ w464]
                          frame Disabled {
                            n285 = flat-sequence {
                              tunnel: w453 -> [w457]
                              tunnel: [w456] -> w454
                              tunnel: w451 -> [w455]
                              tunnel: w454 -> [w458]
                              tunnel: [w458] -> w452
                              frame #0 {
                                n286 = call "CRYUpdate Edit Step Name.vi"("Proper VI No"=w455, "Tree reference In"=w457) -> ("reference out"=w456:refnum<vi>)  [unwired: 9 in]
                              }
                              frame #1 {
                                n287 = call "CRYTS Step Select.vi"("Tree reference In"=w458) -> ("nData_Out"=w460:i32, "sData_Out"=w459:string)  [unwired: 9 out]
                                n288 = call "CRYStep Setup Replace.vi"("Current Step Setup VI No"=w460, "Category"=w459) -> ()  [unwired: 2 in, 8 out]
                              }
                              frame #2 {
                                n289 = call "CRYProject Editor PIC Action End.vi"() -> ()  [unwired: 12 in]
                              }
                            }
                          }
                          frame Enabled {
                            n290 = flat-sequence {
                              tunnel: w466 -> [w472]
                              tunnel: [w472] -> w467
                              tunnel: w464 -> [w471]
                              tunnel: [w471] -> w463
                              tunnel: w462 -> [w468]
                              tunnel: [w468] -> w461
                              tunnel: w467 -> [w475]
                              tunnel: [w475] -> w465
                              tunnel: w463 -> [w474]
                              tunnel: w461 -> [w473]
                              frame #0 {
                                n291 = global read "CRYProject Editor Global.vi" "TS Array"() -> (w469:T7)
                                n292 = Bundle By Name(cluster=w469, "EditStepNo"=w468) -> (w470:T7)
                                n293 = global write "CRYProject Editor Global.vi" "TS Array"(w470) -> ()
                              }
                              frame #1 {
                                n294 = call "CRYStep Setup Replace.vi"("Current Step Setup VI No"=w473, "Category"=w474) -> ()  [unwired: 2 in, 8 out]
                              }
                              frame #2 {
                                n295 = call "CRYProject Editor PIC Action End.vi"() -> ()  [unwired: 12 in]
                              }
                            }
                          }
                        }
                      }
                    }
                  }
                  frame "MoveByVINo" {
                    n296 = call "CRYUpdate Tree for Load.vi"("Is Move?"=TRUE, "ProjectViewCluster In"=w478, "RefTree In"=w479) -> ("RefTree Out"=w476:refnum<vi>)  [unwired: 8 in]
                  }
                  frame "CurLibUpdate" {
                  }
                  frame "ProjectStateChange" {
                  }
                  frame "SelectView" {
                    # "Insert auto select"
                  }
                  frame "SaveStepView" {
                    n297 = call "CRYStep Pic Save SetupView .vi"("nIDV"=w484, "sStepName"=w485) -> ()  [unwired: 10 in]
                  }
                  frame "LoadDisplayStep" {
                    n298 = flat-sequence {
                      tunnel: w490 -> [w494]
                      tunnel: [w495] -> w491
                      tunnel: w489 -> [w495]
                      tunnel: [w492] -> w487
                      tunnel: w491 -> [w498]
                      tunnel: [w496] -> w488
                      tunnel: w487 -> [w496]
                      tunnel: [w503] -> w486
                      tunnel: w488 -> [w503]
                      frame #0 {
                        n299 = call "CRYUpdate Tree for Load.vi"("Is Move?"=FALSE, "ProjectViewCluster In"=w495, "RefTree In"=w494) -> ("RefTree Out"=w492:refnum<vi>)  [unwired: 8 in]
                      }
                      frame #1 {
                        n300 = Unbundle By Name(w498) -> ("Arg1"=w502:string, "Proper VI No"=w501:i32, "Arg2"=w500:string, "Arg3"=w499:string)
                        n301 = call "CRYStep Update.vi"("StepName"=w499, "Step Name Write"=TRUE ("Name/Identifier"), "Seq-step setup"=w500, "Proper VI No"=w501, "StepIdentifier"=w502) -> ()  [unwired: 2 in, 5 out]
                      }
                      frame #2 {
                        n302 = call "CRYProject Editor PIC Action End.vi"() -> ()  [unwired: 12 in]
                      }
                    }
                  }
                  frame "SaveDisplayStep" {
                    w512 = "Display" ("Step File Name")
                    n303 = global read "CRYMainGlobal.vi" "Steps path"() -> (w510:path)
                    n304 = Unbundle By Name(w513) -> ("Arg1"=w505:string, "Proper VI No"=w506:i32)
                    n305 = Build Path(base path=w510, name or relative path="CRYDisplay") -> (appended path=w511:path)
                    n306 = call "CRYStep Write.vi"("StepIdentifier"="", "Default"=FALSE, "Proper VI No"=w506, "Category Name"=w512, "Step File Path"=w511, "Step flattened"=w505, "Step File Name"=w512) -> ()  [unwired: 1 in, 4 out]
                  }
                }
              }
              frame #2 {
                n307 = global read "CRYProject Editor Global.vi" "TS Array"() -> (w523:T7)
                n308 = Unbundle By Name(w520) -> ("Mode"=w519:string, "Ref Variant"=w518:variant, "AllChangeFlg"=w516:bool)
                n309 = Unbundle By Name(w523) -> ("Change State"=w522:bool)
                n310 = control-ref of="TS Tree1"() -> (w514:refnum<vi>)
                n311 = local write "AllChange"(TRUE ("AllChange")) -> ()
                n312 = case shown="\"BooleanWaitingMode\"" w519 {
                  tunnel: w518 -> [w527 _]
                  frame "BooleanWaitingMode" {
                    n313 = Variant To Data(type=refnum<vi> refnum ("Bool Refnum"), Variant=w527) -> (data=w525:refnum<vi>)  [unwired: 1 in, 1 out]
                    n314 = property class="Bool"(reference=w525, "Value"=TRUE ("AllChange")) -> ()  [unwired: 1 in, 2 out]
                  }
                  frame Default {
                  }
                }
                n315 = case shown="False" w522 {
                  frame False {
                    n316 = property on="ProjectStateChange" class="Bool (strict)"("Val(Sgnl)"=TRUE ("Value (Signaling)")) -> ()  [unwired: 2 in, 2 out]
                  }
                  frame True {
                  }
                }
                n317 = control-ref of="This VI"() -> (w515:refnum<vi>)
                n318 = call "CRYUpdate Project Control State.vi"("VI Ref"=w515, "RefTree In"=w514) -> ()  [unwired: 8 in, 2 out]
              }
              frame #3 {
                n319 = local write "bWait"(FALSE ("Project Exist?")) -> ()
                n320 = case shown="True" w530 {
                  tunnel: w529 -> [_ w532]
                  frame False {
                  }
                  frame True {
                    n321 = property on="AllChange" class="Bool (strict)"("Val(Sgnl)"=w532) -> ()  [unwired: 2 in, 2 out]
                  }
                }
              }
            }
          }
          frame True {
          }
        }
      }
    }
    n322 = control-ref of="Pane 3"() -> (w81:refnum<vi>)
    n323 = local read "OldPos"() -> (w82:T1)
    n324 = property class="Pane"(reference=w81) -> ("Bounds"=w77:T1)  [unwired: 1 in, 2 out]
    n325 = Not Equal?(x=w82, y=w77) -> (x != y?=w80:cluster{"Width":bool, "Height":bool})
    n326 = Unbundle By Name(w80) -> ("Width"=w79:bool, "Height"=w78:bool)
    n327 = Or(x=w79, y=w78) -> (x .or. y?=w76:bool)
    n328 = case shown="True" w76 {
      tunnel: w77 -> [_ w109]
      frame False {
      }
      frame True {
        n329 = control-ref of="Pane 3"() -> ()  [unwired: 1 out]
        n330 = local write "OldPos"(w109) -> ()
      }
    }
    n331 = global read "CRYMain Sub Window Global.vi" "gStop"() -> (w86:bool)
    n332 = Or(x=w86, y="stop") -> (x .or. y?=w84:bool)
    n333 = control-ref of="TS Tree1"() -> (w68:refnum<vi>)
    n334 = Build Array("Move Down", "Move Up", "Remove", "Property step", "Property seq", "Add Step") -> (w75:bool[])
    n335 = Search 1D Array(1D array=w75, element=TRUE) -> (index of element=w69:i32)  [unwired: 1 out]
    n336 = case shown="2" w69 {
      tunnel: w68 -> [w89 w95 _ w102 w106 _ _]
      frame 0 {
        n337 = flat-sequence {
          tunnel: [w91] -> w90
          tunnel: w89 -> [w91]
          tunnel: w90 -> [w92]
          frame #0 {
            n338 = call "CRYTS Step Move Down.vi"("Sequence"=w91) -> ()  [unwired: 2 in, 9 out]
          }
          frame #1 {
            n339 = disable-structure shown="Disabled" {
              frame Disabled {
                n340 = call "CRYProject Editor PIC Action End.vi"() -> ()  [unwired: 12 in]
              }
              frame Enabled {
              }
            }
            n341 = property on="ProjectStateChange" class="Bool (strict)"("Val(Sgnl)"=TRUE ("Value (Signaling)")) -> ()  [unwired: 2 in, 2 out]
            n342 = control-ref of="This VI"() -> (w93:refnum<vi>)
            n343 = call "CRYUpdate Project Control State.vi"("VI Ref"=w93, "RefTree In"=w92) -> ()  [unwired: 8 in, 2 out]
          }
        }
      }
      frame 1 {
        n344 = flat-sequence {
          tunnel: [w97] -> w96
          tunnel: w95 -> [w97]
          tunnel: w96 -> [w98]
          frame #0 {
            n345 = call "CRYTS Step Move Up.vi"("TreeRefereneIn"=w97) -> ()  [unwired: 2 in, 9 out]
          }
          frame #1 {
            n346 = disable-structure shown="Disabled" {
              frame Disabled {
                n347 = call "CRYProject Editor PIC Action End.vi"() -> ()  [unwired: 12 in]
              }
              frame Enabled {
              }
            }
            n348 = property on="ProjectStateChange" class="Bool (strict)"("Val(Sgnl)"=TRUE ("Value (Signaling)")) -> ()  [unwired: 2 in, 2 out]
            n349 = control-ref of="This VI"() -> (w99:refnum<vi>)
            n350 = call "CRYUpdate Project Control State.vi"("VI Ref"=w99, "RefTree In"=w98) -> ()  [unwired: 8 in, 2 out]
          }
        }
      }
      frame 2 {
        n351 = property on="StepRemove" class="Bool (strict)"("Val(Sgnl)"=TRUE ("Value (Signaling)")) -> ()  [unwired: 2 in, 2 out]
      }
      frame 3 {
        n352 = call "CRYProject Tree Action Check.vi"("sOption"="Configure", "Project Tree reference"=w102) -> ("bResult"=w103:bool)  [unwired: 8 in, 1 out]
        n353 = case shown="True" w103 {
          tunnel: w102 -> [_ w105]
          frame False {
          }
          frame True {
            n354 = call "CRYConfigure Step.vi"("Project Tree reference"=w105) -> ()  [unwired: 10 in, 1 out]
          }
        }
      }
      frame 4 {
        n355 = call "CRYStart Editor.vi"("Project Tree reference"=w106) -> ()  [unwired: 10 in, 1 out]
      }
      frame 5 {
        n356 = call "CRYAPI WSYSTEM.vi"("sData"="Add Step", "sAction"="OPEN_WIN") -> ()  [unwired: 2 in, 8 out]
      }
      frame Default {
      }
    }
    n357 = control-ref of="This VI"() -> (w83:refnum<vi>)
  }
  n358 = flat-sequence {
    tunnel: w1 -> [w533]
    frame #0 {
      n359 = call "CRYProject LOG OUT.vi"("pVIRef"=w533, "sData"="KILLED:") -> ()  [unwired: 10 in]
    }
    frame #1 {
      w535 = FALSE ("Project Exist?")
      n360 = global write "CRYProject Editor Global.vi" "Expand/Collapse"(w535) -> ()
      n361 = global write "CRYProject Editor Global.vi" "ConfigureShow"(w535) -> ()
      n362 = local write "StateOut"(TRUE ("StateOut")) -> ()
      n363 = global write "CRYProject Editor Global.vi" "Project Exist?"(w535) -> ()
    }
  }
